vi "main_kill_ugshell.vi"   [LabVIEW 2019]
panel:
  # "*******************************************************************\nBiogas Plant Control\n\nAuthor: Paul Zügel\nGCSC-Frankfurt am Main 2020\n\n*******************************************************************"
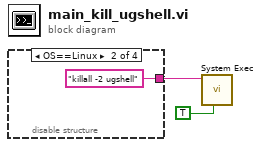
[diagram p0: block diagram]
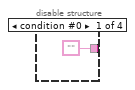
[diagram p2: hidden frame]
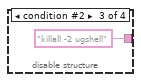
[diagram p3: hidden frame]
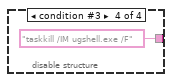
[diagram p4: hidden frame]
diagram:
  n1 = disable-structure shown="OS==Linux" {
    disable-tunnel: ["" "killall -2 ugshell" ("name or relative path") "killall -2 ugshell" ("name or relative path") "taskkill /IM ugshell.exe /F" ("name or relative path")] -> w1
    frame condition #0 {
    }
    frame condition #1 (active) {
    }
    frame condition #2 {
    }
    frame condition #3 {
    }
  }
  n2 = call <vilib>:"System Exec.vi"("run minimized? (F)"=TRUE, "command line"=w1) -> ()  [unwired: 6 in, 4 out]
